vi "Dequeue Packet.vi"(8 "error in (no error)":errorcluster) -> (0 "error out":errorcluster, 1 "Message Data":variant, 2 "Message":enum16{"Error"}(ring), 3 "dup Message Queue":refnum<queue>)   [LabVIEW 2017]
uses:
  Message Cluster.ctl
panel:
  in  "Message Queue":refnum<queue>
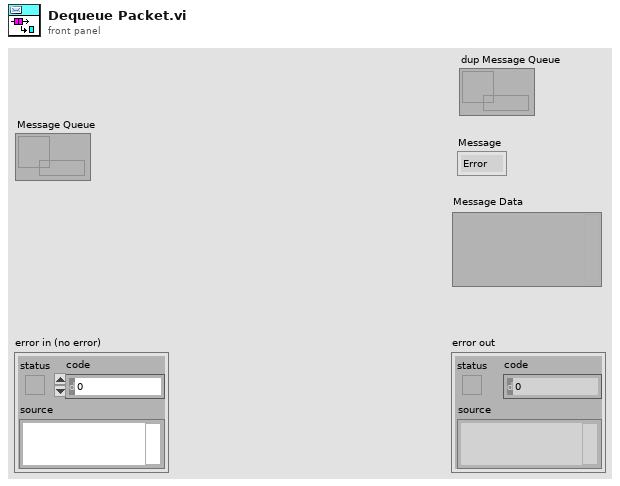
[diagram p1: front panel]
types:
  T1 = typedef "Message Cluster.ctl" = cluster{"Message":enum16{""}, "Message Data":variant}
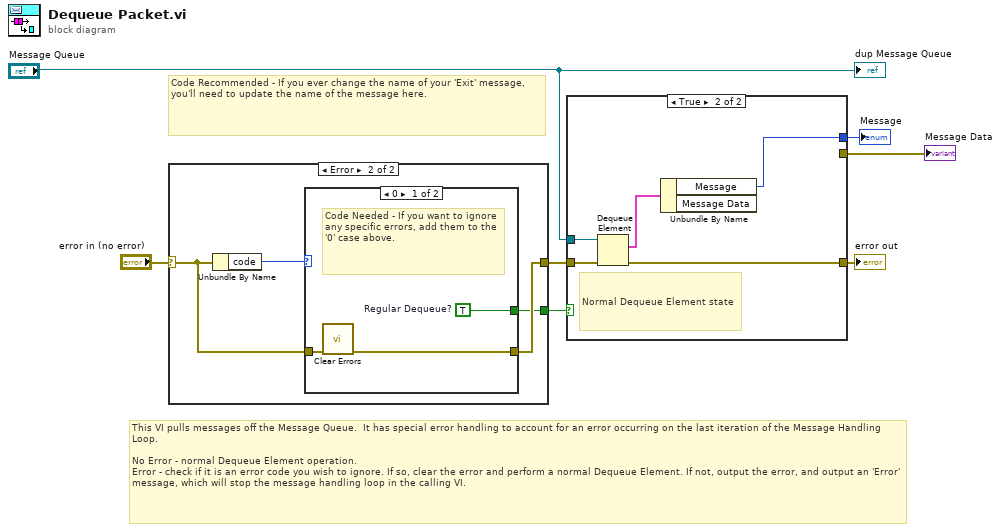
[diagram p0: block diagram]
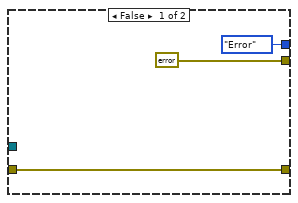
[diagram p2: hidden frame]
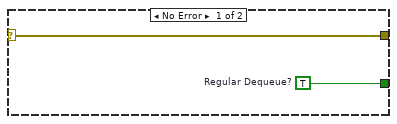
[diagram p3: hidden frame]
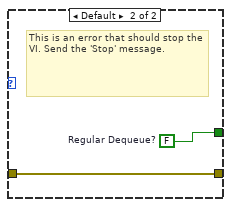
[diagram p4: hidden frame]
diagram:
  # "Code Recommended - If you ever change the name of your 'Exit' message, you'll need to update the name of the message here."
  # "This VI pulls messages off the Message Queue.  It has special error handling to account for an error occurring on the last iteration of the Message Handling Loop.\n\nNo Error - normal Dequeue Element operation.\nError - check if it is an error code you wish to ignore. If so, clear the error and perform a normal Dequeue Element. If not, output the error, and output an 'Error' message, which will stop the message handling loop in the calling VI."
  n1 = case shown="Error" "error in (no error)" {
    selector: "error in (no error)" -> [w9 w12]
    tunnel: [w9 w11] -> w5
    tunnel: [w8 w10] -> w4
    frame No Error {
      w8 = TRUE  # Regular Dequeue?
    }
    frame Error {
      n2 = Unbundle By Name(w12) -> ("code"=w13:i32)
      n3 = case shown="0" w13 {
        tunnel: [w16 w18] -> w11
        tunnel: w12 -> [w15 w18]
        tunnel: [w14 w17] -> w10
        frame 0 {
          w14 = TRUE  # Regular Dequeue?
          # "Code Needed - If you want to ignore any specific errors, add them to the '0' case above."
          n4 = call <vilib>:"Clear Errors.vi"("error in (no error)"=w15) -> ("error out"=w16:errorcluster)  [unwired: 5 in, 1 out]
        }
        frame Default {
          w17 = FALSE  # Regular Dequeue?
          # "This is an error that should stop the VI. Send the 'Stop' message."
        }
      }
    }
  }
  n5 = case shown="True" w4 {
    tunnel: [w21 w26] -> w6
    tunnel: w5 -> [w21 w25]
    tunnel: [errorcluster {"status"=FALSE, "code"=0, "source"=""} ("error IO") _] -> w3
    tunnel: "Message Queue" -> [_ w24]
    tunnel: [enum16{"Error"}."Error" ("Message") w23] -> w2
    frame False {
    }
    frame True {
      # "Normal Dequeue Element state"
      n6 = Dequeue Element(queue=w24, error in (no error)=w25) -> (element=w22:T1, error out=w26:errorcluster)  [unwired: 1 in, 2 out]
      n7 = Unbundle By Name(w22) -> ("Message"=w23:enum16{""})  [unwired: 1 out]
    }
  }
  "error out" <- w6
  "Message Data" <- w3
  "Message" <- w2
  "dup Message Queue" <- "Message Queue"
